vi "get parameter - string.vi"(6 "buffer size (256)":i32=256, 8 "error in (no error)":errorcluster, 10 "parameter":u8 format="%x", 11 "channel":u16 format="%x") -> (0 "error out":errorcluster, 3 "value":string)   [LabVIEW 2024, in "atsj peakcan basic.lvlib"]
doc: "Gets a parameter from a PeakCAN <b>channel</b>."
uses:
  atsj peakcan basic.lvlib
  support/x64/PCANBasic.dll
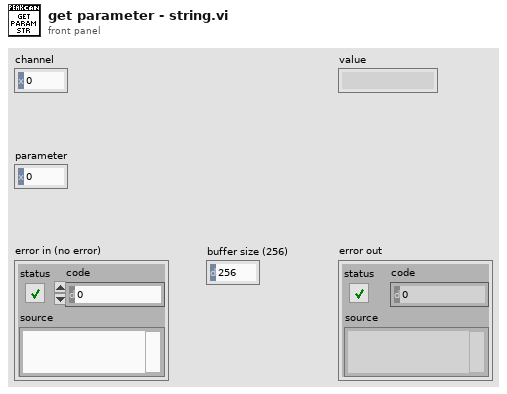
[diagram p1: front panel]
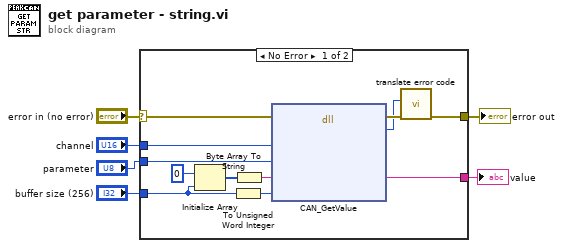
[diagram p0: block diagram]
diagram:
  n1 = case shown="No Error" "error in (no error)" {
    selector: "error in (no error)" -> [w10 w19]
    tunnel: [w11 w19] -> w5
    tunnel: [w12 _] -> w1
    tunnel: "channel" -> [w9 _]
    tunnel: "parameter" -> [w8 _]
    tunnel: "buffer size (256)" -> [w7 _]
    frame No Error {
      n2 = Initialize Array(u8 0, w7) -> (w14:u8[])
      n3 = To Unsigned Word Integer(number=w7) -> (unsigned 16bit integer=w16:u16)
      n4 = Byte Array To String(unsigned byte array=w14) -> (string=w15:string)
      n5 = dll-call lib="C:/atsj/plateau/atsj-peakcan-basic-for-labview/src/support/x64/PCANBasic.dll" fn="CAN_GetValue" ("get parameter - string")(error in=w10, "Channel"=w9, "Parameter"=w8, "Buffer"=w15, "BufferLength"=w16) -> (error out=w18:errorcluster, "Status"=w17:u32, "Buffer"=w12:string)  [unwired: 5 in, 1 out]
      n6 = call "translate error code.vi"("error in (no error)"=w18, "error code"=w17) -> ("error out"=w11:errorcluster)  [unwired: 9 in]
    }
    frame Error {
    }
  }
  "error out" <- w5
  "value" <- w1
